vi "_BroadCastItemKey.vi"(3 "Message":string, 4 "Target":string, 5 "Source":string) -> (2 "Key":string)   [LabVIEW 2014, in "JKI-State-Machine-Plus.lvlib"]
uses:
  JKI-State-Machine-Plus.lvlib
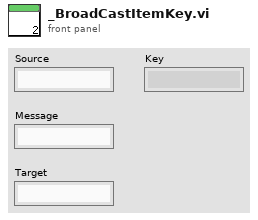
[diagram p1: front panel]
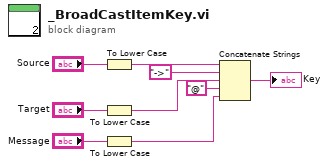
[diagram p0: block diagram]
diagram:
  n1 = To Lower Case(string="Source") -> (all lower case string=w8:string)
  n2 = To Lower Case(string="Target") -> (all lower case string=w2:string)
  n3 = To Lower Case(string="Message") -> (all lower case string=w1:string)
  n4 = Concatenate Strings(w8, "->" ("string"), w2, "@" ("string"), w1) -> (→"Key":string)
